vi "cgi get raw file.vi"(7 "Content-type (\"application/octet-stream\")":string="application/octet-stream", 8 "error in (no error)":errorcluster, 9 "Filename (\"\")":string, 10 "Content (\"\")":string, 11 "HTTP Header (\"\")":string) -> (0 "error out":errorcluster, 2 "Packed Content":string, 3 "HTTP Header":string)   [LabVIEW 2011]
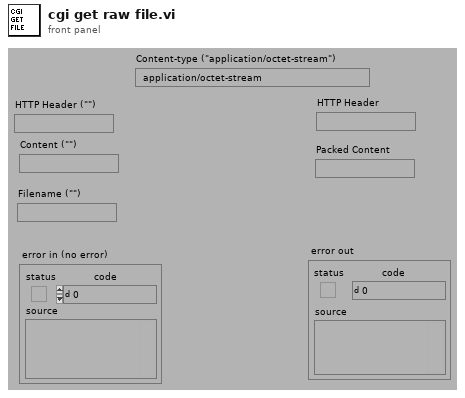
[diagram p1: front panel]
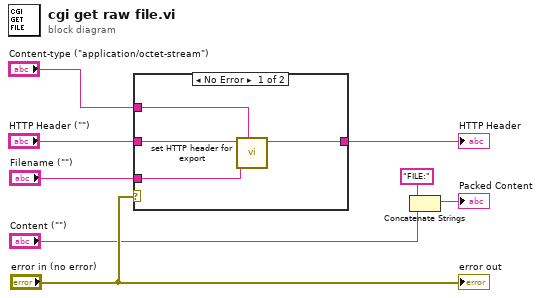
[diagram p0: block diagram]
diagram:
  n1 = case shown="No Error" "error in (no error)" {
    tunnel: "HTTP Header (\"\")" -> [w12 w13]
    tunnel: [w11 w13] -> w4
    tunnel: "Filename (\"\")" -> [w10 _]
    tunnel: "Content-type (\"application/octet-stream\")" -> [w9 _]
    frame No Error {
      n2 = call "set HTTP header for export.vi"("Content-type (\"application/octet-stream\")"=w9, "filename (\"\")"=w10, "HTTP Header (\"\")"=w12) -> ("HTTP Header"=w11:string)  [unwired: 8 out]
    }
    frame Error {
    }
  }
  "HTTP Header" <- w4
  n3 = Concatenate Strings("FILE:" ("Template (\"\")"), "Content (\"\")") -> (→"Packed Content":string)
  "error out" <- "error in (no error)"
